vi "Apply Template if needed.vi"(8 "error in (no error)":errorcluster, 9 "Rest of Input String":string, 10 "From File":string, 11 "Template":string) -> (0 "error out":errorcluster, 2 "Template Applied":bool, 3 "<JSON>":string)   [LabVIEW 2020, in "Config File.lvclass"]
uses:
  <vilib>/JDP Science/JSONtext/Config Files/Config File.lvclass
  <vilib>/Utility/error.llb/Error Cluster From Error Code.vi
  <vilib>/JDP Science/JSONtext/JSONtext.lvlib
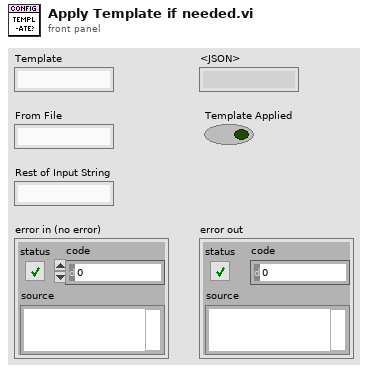
[diagram p1: front panel]
types:
  T1 = typedef "JSONtext.lvlib/JSON Value Type.ctl" = enum16{"Not a JSON Value", "JSON Object", "JSON Array", "String", "Number", "true", "false", "null"}
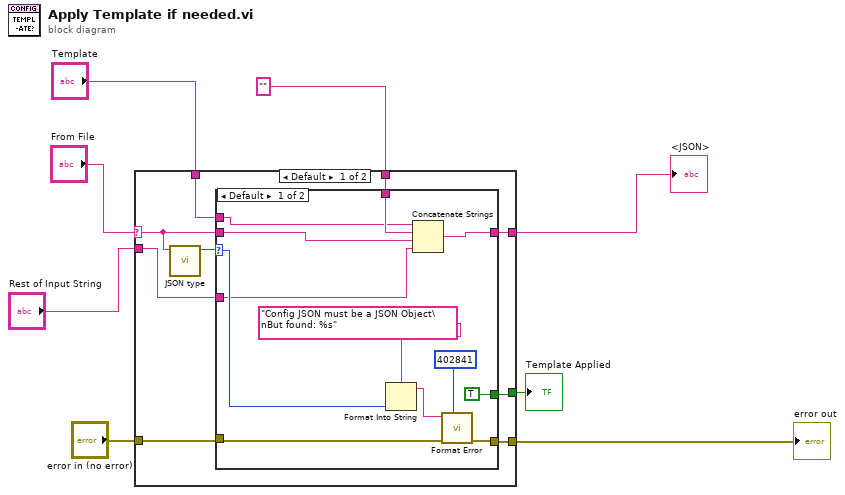
[diagram p0: block diagram]
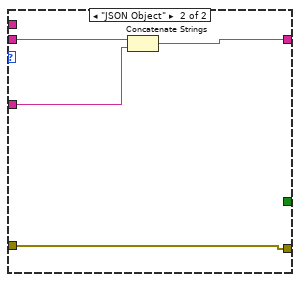
[diagram p2: hidden frame]
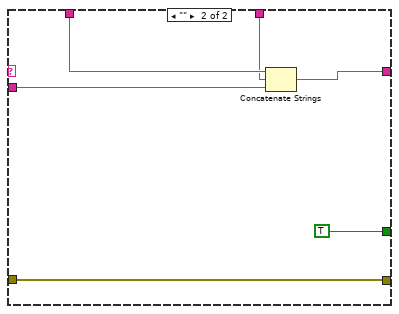
[diagram p3: hidden frame]
diagram:
  n1 = case shown="Default" "From File" {
    selector: "From File" -> [w15 _]
    tunnel: [w16 w38] -> w2
    tunnel: "Template" -> [w14 w39]
    tunnel: "Rest of Input String" -> [w11 w37]
    tunnel: "error in (no error)" -> [w13 w35]
    tunnel: [w12 w35] -> w6
    tunnel: "" ("string") -> [w10 w36]
    tunnel: [w9 TRUE] -> w8
    frame Default {
      n2 = call <vilib>:"JSON type.vi"("JSON"=w15) -> ("JSON Value Type"=w17:T1)  [unwired: 9 in, 1 out]
      n3 = case shown="Default" w17 {
        selector: w17 -> [w24 _]
        tunnel: [w23 w32] -> w16
        tunnel: w15 -> [w20 w33]
        tunnel: w14 -> [w21 _]
        tunnel: w13 -> [w28 w30]
        tunnel: [w29 w30] -> w12
        tunnel: w11 -> [w19 w31]
        tunnel: w10 -> [w22 _]
        tunnel: [TRUE _] -> w9
        frame Default {
          n4 = Format Into String(format string="Config JSON must be a JSON Object\nBut found: %s" ("error message"), w24) -> (resulting string=w26:string)  [unwired: 2 in, 1 out]
          n5 = Concatenate Strings(w21, w22, w20, w19) -> (w23:string)
          n6 = call <vilib>:"Format Error.vi"("error code (402842)"=402841, "error in (no error)"=w28, "error message"=w26) -> ("error out"=w29:errorcluster)  [unwired: 8 in]
        }
        frame "JSON Object" {
          n7 = Concatenate Strings(w33, w31) -> (w32:string)
        }
      }
    }
    frame "" {
      n8 = Concatenate Strings(w39, w36, w37) -> (w38:string)
    }
  }
  "Template Applied" <- w8
  "error out" <- w6
  "<JSON>" <- w2
